vi "reset Cyclone.vi"(8 "error in":errorcluster, 10 "resetDelayInMs":u32, 11 "cycloneHandle":u32) -> (0 "error out":errorcluster, 3 "function return":bool)   [LabVIEW 2021, in "CycloneControlSDK.lvlib"]
doc: "extern \"C\" bool _cdecl resetCyclone(uint32_t cycloneHandle, uint32_t resetDelayInMs);"
uses:
  CycloneControlSDK.lvlib
  CycloneControlSDK_64.dll
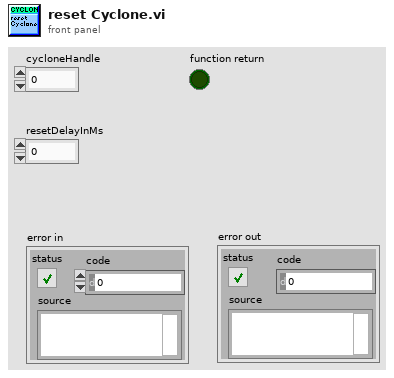
[diagram p1: front panel]
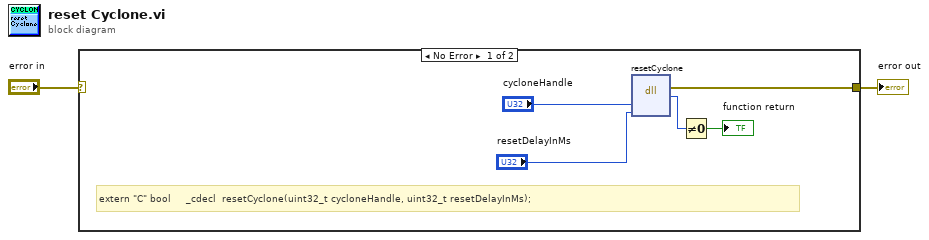
[diagram p0: block diagram]
diagram:
  n1 = case shown="No Error" "error in" {
    selector: "error in" -> [_ w8]
    tunnel: [w3 w8] -> w1
    frame No Error {
      # "extern \"C\" bool     _cdecl  resetCyclone(uint32_t cycloneHandle, uint32_t resetDelayInMs);"
      n2 = dll-call lib="C:/PEMicro/cyclone/cycloneControl/controlsdk/examples/labview2018/user.lib/CycloneControlSDK/CycloneControlSDK_64.dll" fn="resetCyclone"("cycloneHandle"="cycloneHandle", "resetDelayInMs"="resetDelayInMs") -> (error out=w3:errorcluster, "return type"=w6:u8)  [unwired: 5 in, 1 out]
      n3 = Not Equal To 0?(x=w6) -> (x != 0?=→"function return":bool)
    }
    frame Error {
    }
  }
  "error out" <- w1
